vi "test Read Project File.vi"(8 "Error In":errorcluster) -> (0 "Error Out":errorcluster)   [LabVIEW 2015, in "unit tests.lvlib"]
uses:
  unit tests.lvlib
  <vilib>/addons/_JKI Toolkits/Caraya/classes/Assert/Assert False.vi
  <vilib>/addons/_JKI Toolkits/Caraya/classes/Assert/Assert True.vi
  <vilib>/addons/_JKI Toolkits/Caraya/classes/Test/Test.lvclass
  <vilib>/addons/_JKI Toolkits/Caraya/classes/Assert/Assert.lvclass
  LV Project Version Check.lvlib
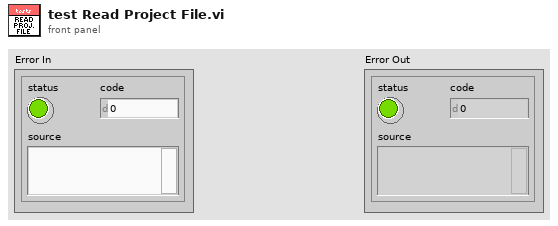
[diagram p1: front panel]
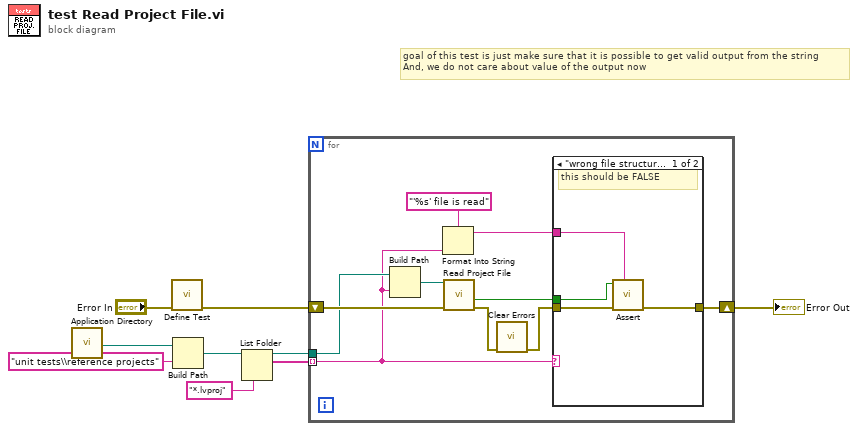
[diagram p0: block diagram]
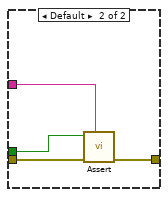
[diagram p2: hidden frame]
diagram:
  # "goal of this test is just make sure that it is possible to get valid output from the string\nAnd, we do not care about value of the output now"
  n1 = call <vilib>:"Application Directory.vi"() -> ("Application Directory"=w8:path)
  n2 = call <vilib>:"Define Test.vi"("error in (no error)"="Error In") -> ("error out"=w4:errorcluster)  [unwired: 10 in]
  n3 = Build Path(base path=w8, name or relative path="unit tests\\reference projects") -> (appended path=w6:path)
  n4 = List Folder(path=w6, pattern="*.lvproj") -> (path out=w1:path, filenames=w2:string[])  [unwired: 2 in, 2 out]
  n5 = for {
    shift-right: [w19] -> w3
    shift-left: w4 -> [w18]
    tunnel: w2 -> [w11] mode=indexing
    tunnel: w1 -> [w17]
    n6 = Build Path(base path=w17, name or relative path=w11) -> (appended path=w14:path)
    n7 = Format Into String(format string="'%s' file is read", w11) -> (resulting string=w13:string)  [unwired: 2 in, 1 out]
    n8 = call "Read Project File.vi"("Error In"=w18, "path to XML document"=w14) -> ("Error Out"=w16:errorcluster, "Valid?"=w15:bool)  [unwired: 7 in, 1 out]
    n9 = call <vilib>:"Clear Errors.vi"("error in (no error)"=w16) -> ("error out"=w10:errorcluster)  [unwired: 5 in, 1 out]
    n10 = case shown="\"wrong file structure.lvproj\"" w11 {
      tunnel: [w22 w27] -> w19
      tunnel: w10 -> [w23 w26]
      tunnel: w15 -> [w21 w25]
      tunnel: w13 -> [w20 w24]
      frame "wrong file structure.lvproj" {
        # "this should be FALSE"
        n11 = call-poly <vilib>:"Assert.vi"("Label"=w20, "error in (no error)"=w23, "False?"=w21) -> ("error out"=w22:errorcluster)  [unwired: 8 in]
      }
      frame Default {
        n12 = call-poly <vilib>:"Assert.vi"("Label"=w24, "error in (no error)"=w26, "True?"=w25) -> ("error out"=w27:errorcluster)  [unwired: 8 in]
      }
    }
  }
  "Error Out" <- w3
